vi "Peer To Peer Reader - Basic (FPGA).vi"() -> ()   [LabVIEW 2018]
uses:
  <vilib>/Platform/TimedLoop/XDataNode/timing_clust.ctl
  <vilib>/Platform/TimedLoop/XDataNode/nitl_modes.ctl
  <vilib>/Platform/TimedLoop/XDataNode/wakeup.ctl
  <vilib>/rvi/Emulation/niFpgaSctlEmulationGetInTimedLoop.vi
  <vilib>/rvi/Emulation/niFpgaEmulationReportErrorSimple.vi
  <vilib>/rvi/Emulation/niFpgaGetClockAttributes.vi
  <vilib>/rvi/Emulation/niFpgaCriticalErrorInLSC.vi
  <vilib>/Platform/TimedLoop/XDataNode/XDataNode.xnode
  <vilib>/rvi/DataTransferAndStorage/Container/XNode/niFpgaContainer.xnode
  <vilib>/rvi/FIFO/Fifo_Resource/nirvififoEmulationP2P.vi
  <vilib>/Platform/TimedLoop/XDataNode/XDNodeRunTimeDep.lvlib
panel:
  out "Data Valid?":bool
  out "Data Read":u64
  out "Data Expected":u64
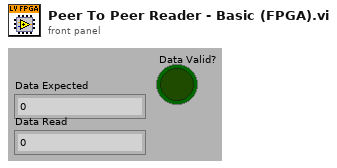
[diagram p1: front panel]
types:
  T1 = typedef "XDNodeRunTimeDep.lvlib/timing_clust.ctl" = cluster{"Expected End [f-1]":u64, "Actual End [f-1]":u64, "Finished Late? [f-1]":bool, "Expected End [i-1]":u64, "Actual End [i-1]":u64, "Finished Late? [i-1]":bool, "Expected Start [i]":u64, "Actual Start [i]":u64, "Expected Start [f]":u64, "Actual Start [f]":u64, "Source Name":string, "Structure Name":string, "Period":i64, "Deadline":i64, "Offset":i64, "Start":i64, "Priority":i32, "Timeout":i32, "Mode":T2, "Wakeup Reason":T3, "Error":errorcluster, "Source Type":string, "Secondary Source Type":string, "Global End Time":u64, "Global Start Time":u64, "Frame Duration":u64, "Iteration Duration":u64, "Assigned CPU":i32, "I/O Scan Engine Mode":u32}
  T2 = typedef "XDNodeRunTimeDep.lvlib/nitl_modes.ctl" = enum32{"No Change", "Process missed periods, maintain original phase", "Discard missed periods, maintain original phase", "Process missed periods, ignore original phase", "Discard missed periods, ignore original phase"}
  T3 = typedef "XDNodeRunTimeDep.lvlib/wakeup.ctl" = enum32{"Normal", "Aborted", "Asynchronous wakeup", "Timing source error", "Timed loop error", "Timeout"}
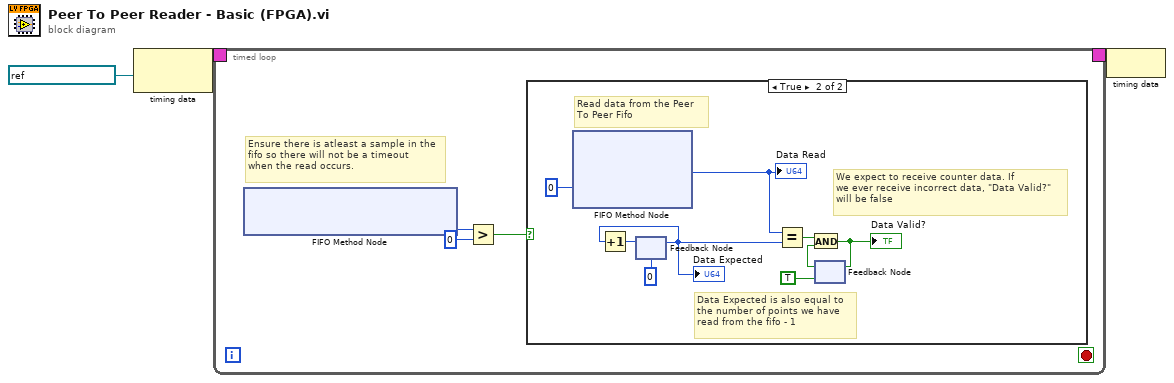
[diagram p0: block diagram]
diagram:
  n1 = node-c288(refnum<k21> "100 MHz Clock" ("Source Name")) -> (w3:T1)
  n2 = timed-loop {
    timing: w3 -> [_]
    timing-out: [_] -> w2
    stop <- _ stop-if-true
    # "Ensure there is atleast a sample in the\nfifo so there will not be a timeout\nwhen the read occurs."
    n3 = xnode ("FIFO Method Node")() -> ("Number of Elements to Read"=w6:u32)  [unwired: 1 in, 1 out]
    n4 = Greater?(x=w6, y=u32 0) -> (0:w4:bool)
    n5 = case shown="True" w4 {
      frame False {
      }
      frame True {
        # "We expect to receive counter data. If \nwe ever receive incorrect data, \"Data Valid?\"\nwill be false"
        # "Data Expected is also equal to\nthe number of points we have\nread from the fifo - 1"
        # "Read data from the Peer \nTo Peer Fifo"
        n6 = xnode ("FIFO Method Node")("Timeout"=0) -> ("Element"=w12:u64)  [unwired: 1 in, 2 out]
        "Data Read" <- w12
        n7 = feedback #1(u64 0 ("Element")) -> (w11:u64)
        "Data Expected" <- w11
        n8 = Increment(x=w11) -> (x+1=w13:u64)
        n9 = feedback-in #1(w13) -> ()
        n10 = Equal?(x=w12, y=w11) -> (x = y?=w10:bool)
        n11 = feedback #2(TRUE) -> (w9:bool)
        n12 = And(x=w10, y=w9) -> (x .and. y?=w7:bool)
        "Data Valid?" <- w7
        n13 = feedback-in #2(w7) -> ()
      }
    }
  }
  n14 = node-c288(w2) -> ()
